vi "Process_data.vi"(2 "error in (no error)":errorcluster, 3 "String to process":string) -> (0 "error out (no error)":errorcluster, 1 "String to send":string)   [LabVIEW 2011]
doc: "Process_data\n\nProcesses and executes the client settings and makes a result packet that will be sent back to the client."
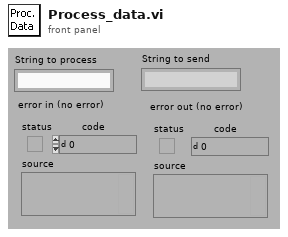
[diagram p1: front panel]
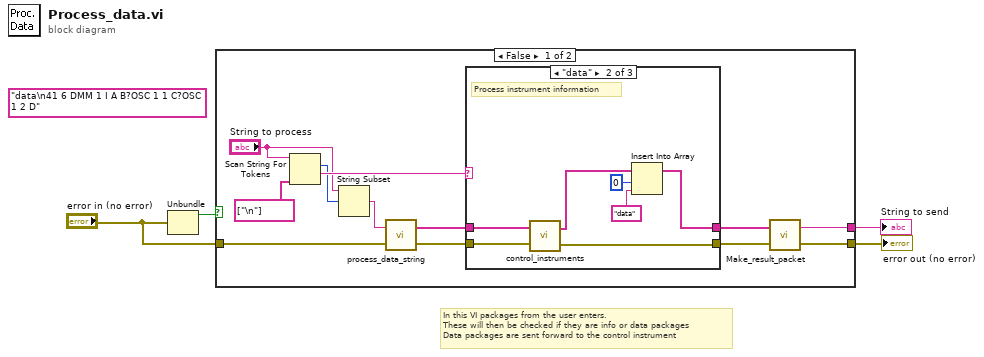
[diagram p0: block diagram]
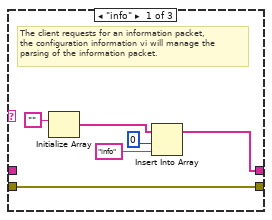
[diagram p2: hidden frame]
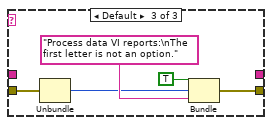
[diagram p3: hidden frame]
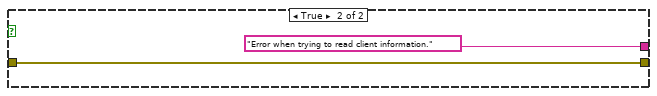
[diagram p4: hidden frame]
diagram:
  (unwired) "data\n41 6 DMM 1 I A B?OSC 1 1 C?OSC 1 2 D"
  # "In this VI packages from the user enters.\nThese will then be checked if they are info or data packages\nData packages are sent forward to the control instrument"
  n1 = Unbundle("error in (no error)") -> ("status"=w2:bool)  [unwired: 2 out]
  n2 = case shown="False" w2 {
    tunnel: [w16 "Error when trying to read client information."] -> w4
    tunnel: [w15 w35] -> w3
    tunnel: "error in (no error)" -> [w14 w35]
    frame False {
      n3 = Scan String For Tokens(6:string[] ["\n"] ("delimiters (\\s,\\t,\\r,\\n)"), 9:"String to process") -> (1:w8:string, 2:w7:i32)  [unwired: 4 in, 2 out]
      n4 = String Subset(string="String to process", offset (0)=w7) -> (substring=w9:string)  [unwired: 1 in]
      n5 = call "process_data_string.vi"("error in (no error)"=w14, "Data in"=w9) -> ("error out (no error)"=w11:errorcluster, "Data out"=w13:string[])
      n6 = case shown="\"data\"" w8 {
        tunnel: w13 -> [_ w29 _]
        tunnel: [w22 w27 w31] -> w12
        tunnel: w11 -> [w22 w28 w30]
        tunnel: [w21 w24 _] -> w10
        frame "info" {
          # "The client requests for an information packet,\nthe configuration information vi will manage the\nparsing of the information packet."
          n7 = Initialize Array("" ("element")) -> (w18:string[])  [unwired: 1 in]
          n8 = Insert Into Array(array=w18, index=0, new element="info") -> (w21:string[])
        }
        frame "data" {
          # "Process instrument information"
          n9 = call "control_instruments.vi"("error in (no error)"=w28, "Data in"=w29) -> ("error out (no error)"=w27:errorcluster, "Measurement Data"=w23:string[])
          n10 = Insert Into Array(array=w23, index=0, new element="data" ("new element/subarray")) -> (w24:string[])
        }
        frame Default {
          n11 = Unbundle(w30) -> ("code"=w32:i32)  [unwired: 2 out]
          n12 = Bundle("status"=TRUE, "code"=w32, "Process data VI reports:\nThe first letter is not an option.") -> (w31:cluster{"status":bool, "code":i32, string})  [unwired: 1 in]
        }
      }
      n13 = call "Make_result_packet.vi"("error in (no error)"=w12, "Measuredata in"=w10) -> ("error out (no error)"=w15:errorcluster, "String to Send"=w16:string)
    }
    frame True {
    }
  }
  "String to send" <- w4
  "error out (no error)" <- w3
